vi "Control loop.vi"(8 "error in (no error)":errorcluster) -> ()   [LabVIEW 2011]
uses:
  point.ctl
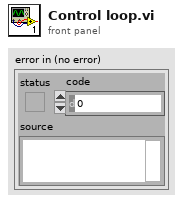
[diagram p1: front panel]
types:
  T1 = enum16{"Startup", "Run program", "Home", "Hold position", "Stop"}
  T2 = typedef "point.ctl" = cluster{"X":dbl, "Y":dbl, "Z":dbl, "Ramp":dbl, "Speed":dbl}
  T3 = enum16{"Startup", "Run program", "Home", "Hold position"}
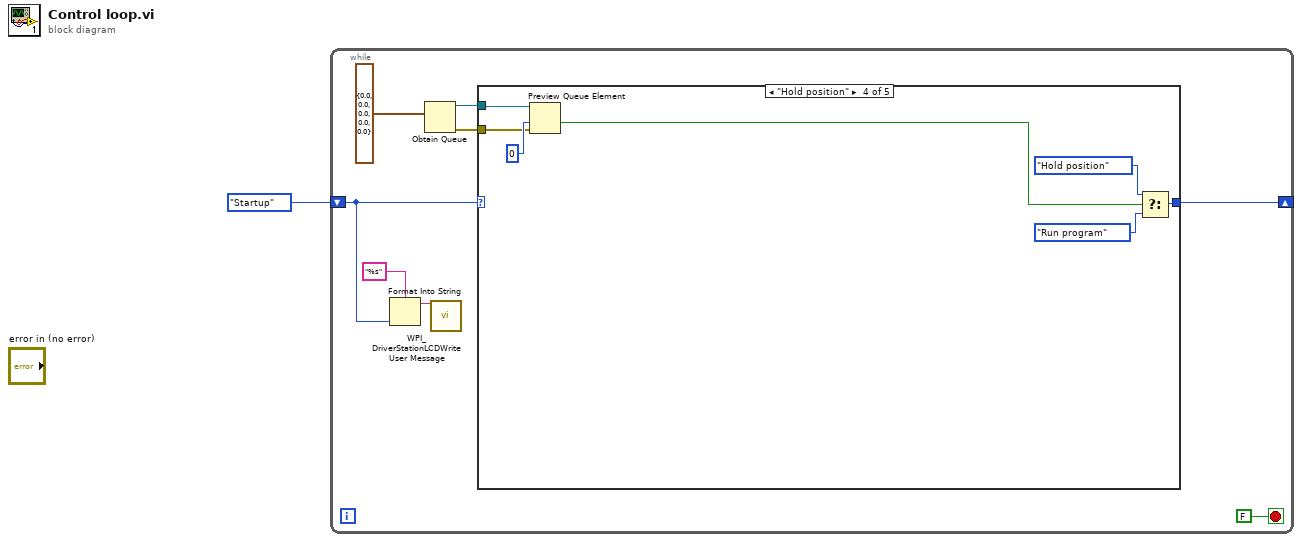
[diagram p0: block diagram]
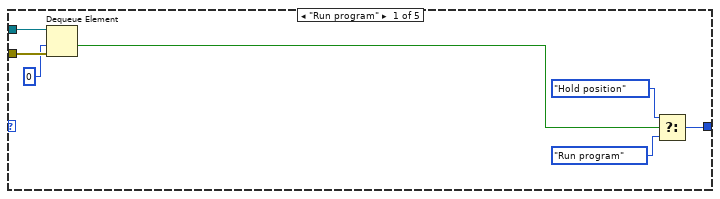
[diagram p2: hidden frame]
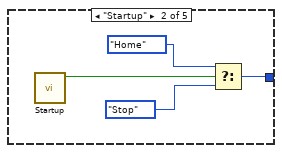
[diagram p3: hidden frame]
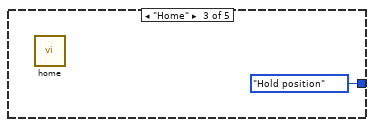
[diagram p4: hidden frame]
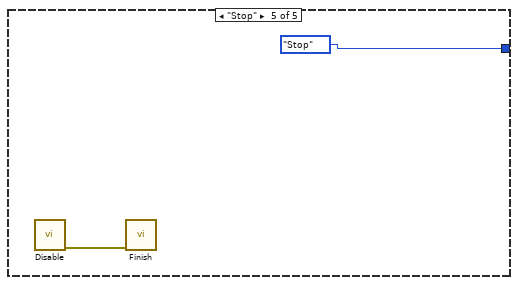
[diagram p5: hidden frame]
diagram:
  n1 = while {
    shift-right: [w7] -> _
    shift-left: T1."Startup" ("Enum") -> [w4]
    stop <- FALSE stop-if-true
    n2 = Format Into String(format string="%s", w4) -> (resulting string=w2:string)  [unwired: 2 in, 1 out]
    n3 = Obtain Queue(element data type=T2 {"X"=0.0, "Y"=0.0, "Z"=0.0, "Ramp"=0.0, "Speed"=0.0} ("Point")) -> (queue out=w6:refnum<queue>, error out=w5:errorcluster)  [unwired: 4 in, 1 out]
    n4 = call <vilib>:"WPI_DriverStationLCDWrite User Message.vi"("line text"=w2) -> ()  [unwired: 14 in, 1 out]
    n5 = case shown="\"Hold position\"" w4 {
      tunnel: [w13 w19 T3."Hold position" w24 T1."Stop" ("Enum")] -> w7
      tunnel: w6 -> [w16 _ _ w23 _]
      tunnel: w5 -> [w15 _ _ w22 _]
      frame "Run program" {
        n6 = Dequeue Element(queue=w16, timeout in ms (-1)=0, error in (no error)=w15) -> (timed out?=w10:bool)  [unwired: 3 out]
        n7 = Select(t=T3."Hold position", s=w10, f=T3."Run program") -> (s? t:f=w13:T3)
      }
      frame "Startup" {
        n8 = call "Startup.vi"() -> ("Good"=w20:bool)  [unwired: 11 in]
        n9 = Select(t=T3."Home", s=w20, f=T1."Stop" ("Enum")) -> (s? t:f=w19:T1)
      }
      frame "Home" {
        n10 = call "home.vi"() -> ()  [unwired: 12 in]
      }
      frame "Hold position" {
        n11 = Preview Queue Element(queue=w23, timeout in ms (-1)=0, error in (no error)=w22) -> (timed out?=w25:bool)  [unwired: 3 out]
        n12 = Select(t=T3."Hold position", s=w25, f=T3."Run program") -> (s? t:f=w24:T3)
      }
      frame "Stop" {
        n13 = call "Disable.vi"() -> ("error out"=w29:errorcluster)  [unwired: 11 in]
        n14 = call "Finish.vi"("error in (no error)"=w29) -> ()  [unwired: 10 in, 1 out]
      }
    }
  }
